vi "FindStats.vi"(11 "Actor.lvclass":variant) -> (3 "Stats":T1)   [LabVIEW 2020, in "jettl.lvlib"]
uses:
  jettl.lvlib
  Msg/Msg.lvclass
  MsgSet.ctl
  <vilib>/Utility/Data Type/NI_Data Type.lvlib
  Stats.ctl
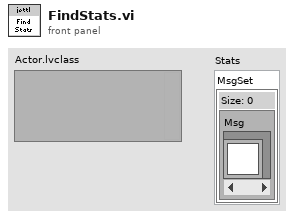
[diagram p1: front panel]
types:
  T1 = typedef "jettl.lvlib/Stats.ctl" = cluster{"MsgSet":T2}
  T2 = typedef "jettl.lvlib/MsgSet.ctl" = set{refnum<class "Msg.lvclass">}
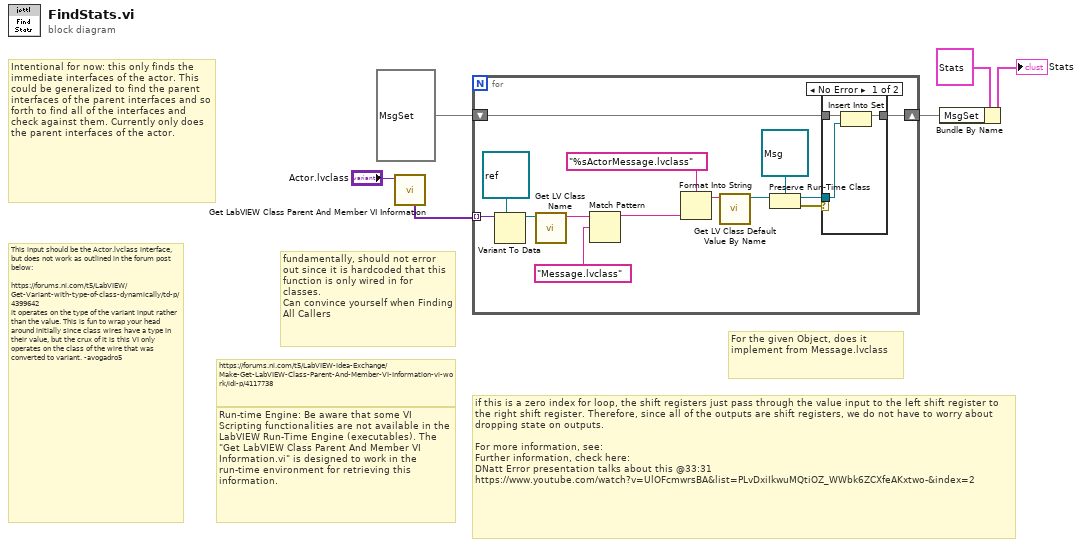
[diagram p0: block diagram]
diagram:
  # "fundamentally, should not error out since it is hardcoded that this function is only wired in for classes.\nCan convince yourself when Finding All Callers"
  # "if this is a zero index for loop, the shift registers just pass through the value input to the left shift register to the right shift register. Therefore, since all of the outputs are shift registers, we do not have to worry about dropping state on outputs.\n\nFor more information, see:\nFurther information, check here:\nDNatt Error presentation talks about this @33:31\nhttps://www.youtube.com/watch?v=UlOFcmwrsBA&list=PLvDxiIkwuMQtiOZ_WWbk6ZCXfeAKxtwo-&index=2"
  # "For the given Object, does it implement from Message.lvclass"
  # "This input should be the Actor.lvclass interface, but does not work as outlined in the forum post below:\n\nhttps://forums.ni.com/t5/LabVIEW/Get-Variant-with-type-of-class-dynamically/td-p/4399642\nit operates on the type of the variant input rather than the value. This is fun to wrap your head around initially since class wires have a type in their value, but the crux of it is this VI only operates on the class of the wire that was converted to variant. -avogadro5"
  # "Intentional for now: this only finds the immediate interfaces of the actor. This could be generalized to find the parent interfaces of the parent interfaces and so forth to find all of the interfaces and check against them. Currently only does the parent interfaces of the actor."
  # "Run-time Engine: Be aware that some VI Scripting functionalities are not available in the LabVIEW Run-Time Engine (executables). The \"Get LabVIEW Class Parent And Member VI Information.vi\" is designed to work in the run-time environment for retrieving this information."
  # "https://forums.ni.com/t5/LabVIEW-Idea-Exchange/Make-Get-LabVIEW-Class-Parent-And-Member-VI-Information-vi-work/idi-p/4117738"
  n1 = call <vilib>:"Get LabVIEW Class Parent And Member VI Information.vi"("variant"="Actor.lvclass") -> ("parent interfaces"=w4:variant[])  [unwired: 7 in, 3 out]
  n2 = for {
    tunnel: w4 -> [w19] mode=indexing
    shift-right: [w15] -> w1
    shift-left: T2 {} ("MsgSet") -> [w16]
    n3 = Variant To Data(type=refnum<class> refnum ("LabVIEW Object"), Variant=w19) -> (data=w18:refnum<class>)  [unwired: 1 in, 1 out]
    n4 = call <vilib>:"Get LV Class Name.vi"("object"=w18) -> ("class name"=w9:string)  [unwired: 9 in, 1 out]
    n5 = Match Pattern(string=w9, regular expression="Message.lvclass" ("string")) -> (before substring=w8:string)  [unwired: 1 in, 3 out]
    n6 = Format Into String(format string="%sActorMessage.lvclass", w8) -> (resulting string=w7:string)  [unwired: 2 in, 1 out]
    n7 = call <vilib>:"Get LV Class Default Value By Name.vi"("class name"=w7) -> ("object"=w17:refnum<class>)  [unwired: 9 in, 1 out]
    n8 = Preserve Run-Time Class(object in=w17, 2:refnum<class "Msg.lvclass"> refnum ("Msg")) -> (object out=w12:refnum<class "Msg.lvclass">, error out=w10:errorcluster)  [unwired: 1 in]
    n9 = case shown="No Error" w10 {
      tunnel: w16 -> [w23 w24]
      tunnel: [w22 w24] -> w15
      tunnel: w12 -> [w21 _]
      frame No Error {
        n10 = Insert Into Set(10:w21, 11:w23) -> (3:w22:T2)  [unwired: 1 out]
      }
      frame Error {
      }
    }
  }
  n11 = Bundle By Name(cluster=T1 {"MsgSet"={}} ("Stats"), "MsgSet"=w1) -> (→"Stats":T1)
